vi "DCA Pluck Data for Display.vi"(4 "Measurement Values":T3) -> (0 "Calculated Values":T1, 1 "Measure Values":T2, 2 "Zo (W)":dbl)   [LabVIEW 2011]
uses:
  TypeDefs/DCA Measurement Values.ctl
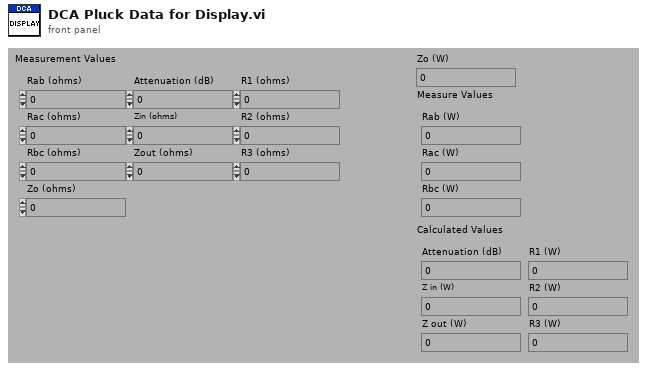
[diagram p1: front panel]
types:
  T1 = cluster{"Attenuation (dB)":dbl, "Z out (W)":dbl, "Z in (W)":dbl, "R1 (W)":dbl, "R2 (W)":dbl, "R3 (W)":dbl}
  T2 = cluster{"Rab (W)":dbl, "Rac (W)":dbl, "Rbc (W)":dbl}
  T3 = typedef "DCA Measurement Values.ctl" = cluster{"Rab (ohms)":dbl, "Rac (ohms)":dbl, "Rbc (ohms)":dbl, "Zo (ohms)":dbl, "Attenuation (dB)":dbl, "Zin (ohms)":dbl, "Zout (ohms)":dbl, "R1 (ohms)":dbl, "R2 (ohms)":dbl, "R3 (ohms)":dbl}
  T4 = cluster{"Rab (ohms)":dbl, "Rac (ohms)":dbl, "Rbc (ohms)":dbl}
  T5 = cluster{"Attenuation (dB)":dbl, "Zin (ohms)":dbl, "Zout (ohms)":dbl, "R1 (ohms)":dbl, "R2 (ohms)":dbl, "R3 (ohms)":dbl}
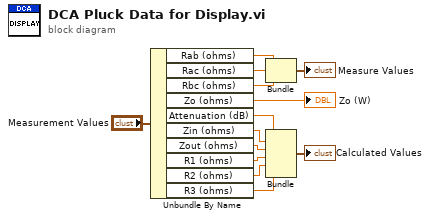
[diagram p0: block diagram]
diagram:
  n1 = Unbundle By Name("Measurement Values") -> ("Rab (ohms)"=w12:dbl, "Rac (ohms)"=w11:dbl, "Rbc (ohms)"=w10:dbl, "Zo (ohms)"=→"Zo (W)":dbl, "Attenuation (dB)"=w8:dbl, "Zin (ohms)"=w6:dbl, "Zout (ohms)"=w4:dbl, "R1 (ohms)"=w3:dbl, "R2 (ohms)"=w5:dbl, "R3 (ohms)"=w7:dbl)
  n2 = Bundle("Rab (ohms)"=w12, "Rac (ohms)"=w11, "Rbc (ohms)"=w10) -> (→"Measure Values":T4)  [unwired: 1 out]
  n3 = Bundle("Attenuation (dB)"=w8, "Zin (ohms)"=w6, "Zout (ohms)"=w4, "R1 (ohms)"=w3, "R2 (ohms)"=w5, "R3 (ohms)"=w7) -> (→"Calculated Values":T5)  [unwired: 1 out]
